vi "Write Path.vi"(8 "error in (no error)":errorcluster, 10 "Path":path, 11 "Logging_Contador_Actor in":refnum<class "Logging_Contador_Actor.lvclass">) -> (0 "error out":errorcluster, 3 "Logging_Contador_Actor out":refnum<class "Logging_Contador_Actor.lvclass">)   [LabVIEW 2019, in "Logging_Contador_Actor.lvlib" / "Logging_Contador_Actor.lvclass"]
uses:
  Logging_Contador_Actor.lvclass
  Logging_Contador_Actor.lvclass/Logging_Contador_Actor.ctl
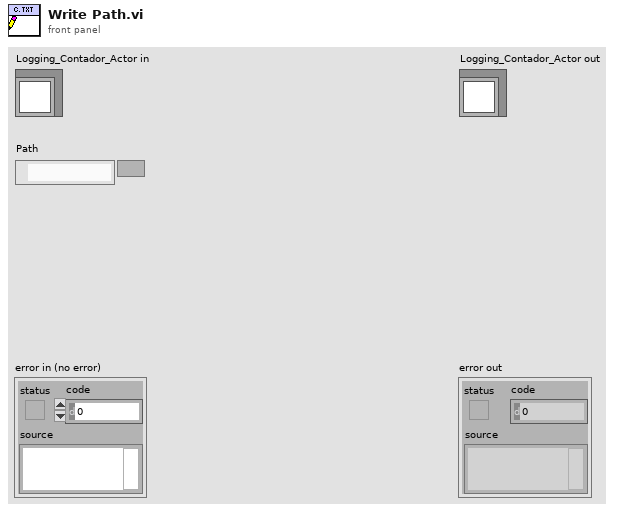
[diagram p1: front panel]
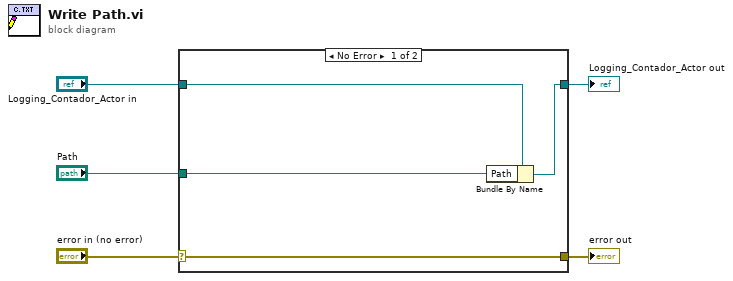
[diagram p0: block diagram]
diagram:
  n1 = case shown="No Error" "error in (no error)" {
    selector: "error in (no error)" -> [w9 w10]
    tunnel: [w9 w10] -> w4
    tunnel: [w7 w11] -> w2
    tunnel: "Logging_Contador_Actor in" -> [w8 w11]
    tunnel: "Path" -> [w6 _]
    frame No Error {
      n2 = Bundle By Name(cluster=w8, "Path"=w6) -> (w7:refnum<class "Logging_Contador_Actor.lvclass">)
    }
    frame Error {
    }
  }
  "error out" <- w4
  "Logging_Contador_Actor out" <- w2
